vi "Setup VI for Full Monitor Res.vi"(8 "Error In":errorcluster, 11 "This VI":refnum<vi>) -> (0 "Error Out":errorcluster, 3 "VI Ref Out":refnum<vi>)   [LabVIEW 2014]
uses:
  <vilib>/Utility/miscctls.llb/LVRectTypeDef.ctl
  <vilib>/Utility/miscctls.llb/LVPointTypeDef.ctl
panel:
  out "Front Panel Window:Panel Bounds":T1
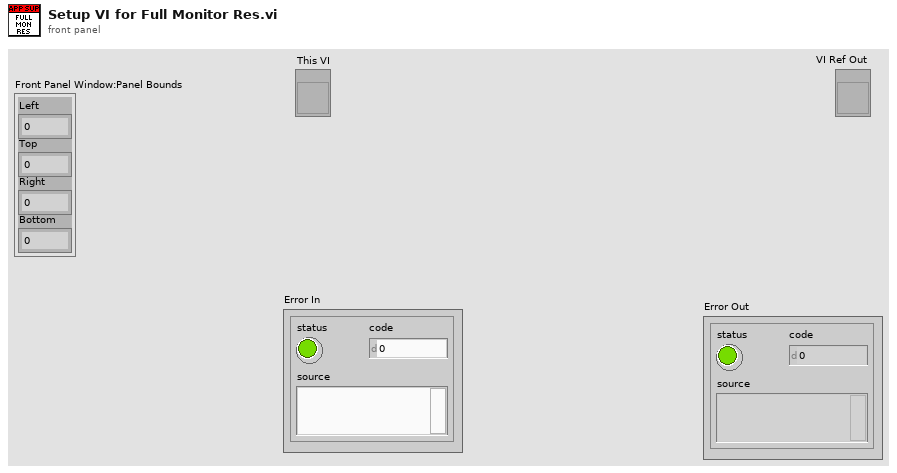
[diagram p1: front panel]
types:
  T1 = typedef "LVRectTypeDef.ctl" = cluster{"Left":i16, "Top":i16, "Right":i16, "Bottom":i16}
  T2 = typedef "LVPointTypeDef.ctl" = cluster{"Horizontal":i16, "Vertical":i16}
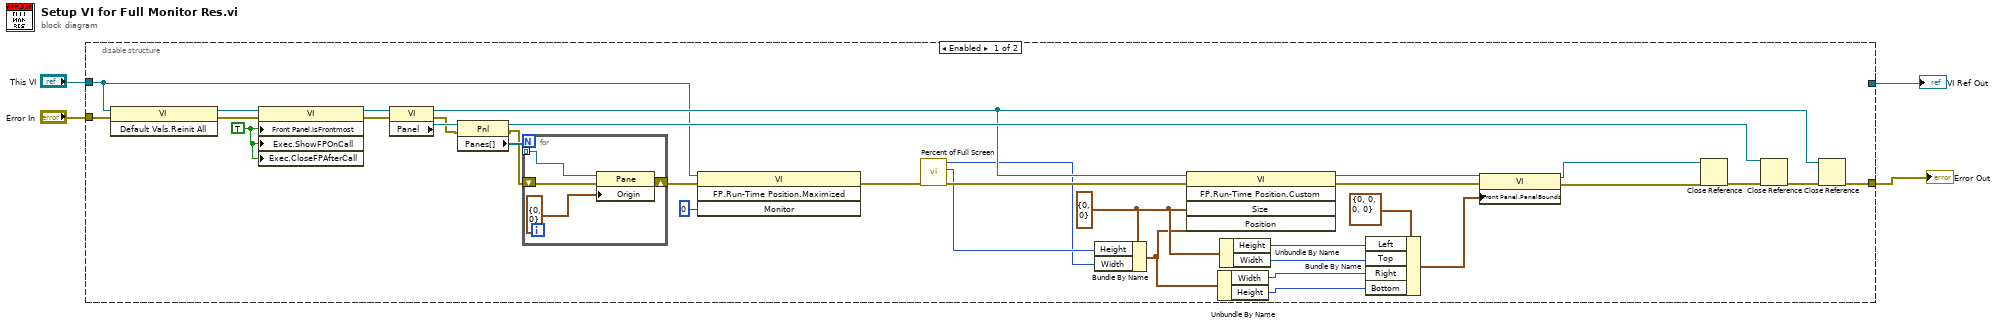
[diagram p0: block diagram]
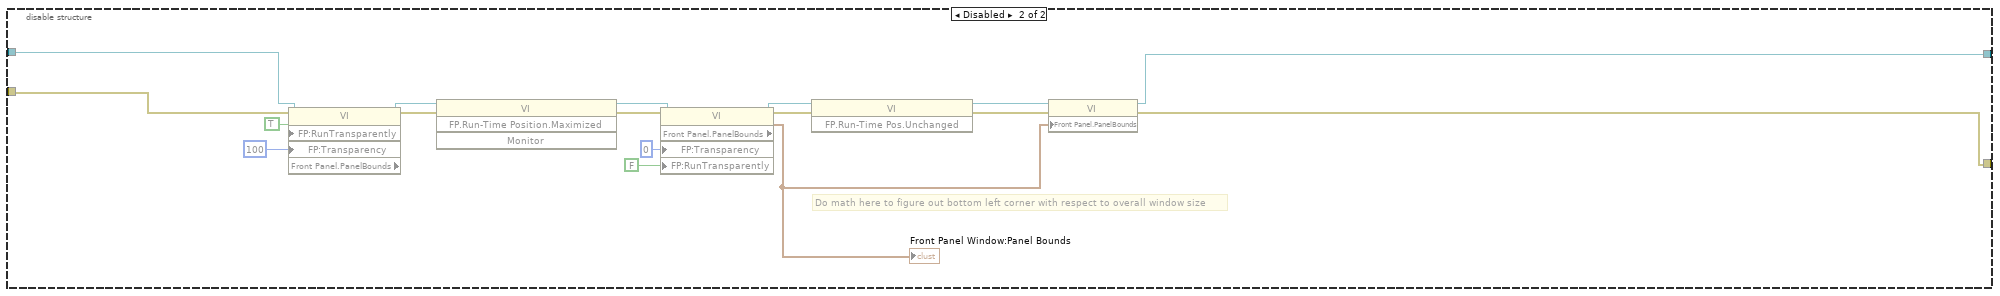
[diagram p2: hidden frame]
diagram:
  n1 = disable-structure shown="Enabled" {
    disable-tunnel: "Error In" -> [w38 w45]
    disable-tunnel: [w30 w43] -> w3
    disable-tunnel: "This VI" -> [w18 w46]
    disable-tunnel: [_ w44] -> w1
    frame Enabled {
      w24 = TRUE ("Front Panel Window:Is Frontmost")
      w11 = cluster{"Height":i16, "Width":i16} {"Height"=0, "Width"=0} ("Size")
      n2 = invoke class="VI" method="Default Vals.Reinit All"(reference=w18, error in=w38) -> (reference out=w28:refnum<vi>, error out=w25:errorcluster)  [unwired: 1 in, 1 out]
      n3 = property on="Property Node" class="VI"(reference=w28, error in=w25, "Front Panel.IsFrontmost"=w24, "Exec.ShowFPOnCall"=w24, "Exec.CloseFPAfterCall"=w24) -> (reference out=w27:refnum<vi>, error out=w26:errorcluster)
      n4 = property on="Property Node" class="VI"(reference=w27, error in=w26) -> (reference out=w29:refnum<vi>, error out=w35:errorcluster, "Panel"=w37:refnum<vi>)
      n5 = property on="Property Node" class="Pnl"(reference=w37, error in=w35) -> (reference out=w32:refnum<vi>, error out=w34:errorcluster, "Panes[]"=w36:refnum<vi>[])
      n6 = for {
        tunnel: w36 -> [w39] mode=indexing
        shift-right: [w40] -> w20
        shift-left: w34 -> [w41]
        n7 = property on="Property Node" class="Pane"(reference=w39, error in=w41, "Origin"=T2 {"Horizontal"=0, "Vertical"=0}) -> (error out=w40:errorcluster)  [unwired: 1 out]
      }
      n8 = invoke class="VI" method="FP.Run-Time Position.Maximized"(reference=w18, error in=w20, "Monitor"=i16 0) -> (error out=w17:errorcluster)  [unwired: 1 in, 3 out]
      n9 = call "Percent of Full Screen.vi"("error in (no error)"=w17) -> ("error out"=w23:errorcluster, "Bottom"=w22:i16, "Right"=w21:i16)  [unwired: 8 in]
      n10 = Bundle By Name(cluster=w11, "Height"=w22, "Width"=w21) -> (w8:cluster{"Height":i16, "Width":i16})
      n11 = invoke class="VI" method="FP.Run-Time Position.Custom"(reference=w29, error in=w23, "Size"=w11, "Position"=w8) -> (reference out=w16:refnum<vi>, error out=w15:errorcluster)  [unwired: 1 in, 3 out]
      n12 = Unbundle By Name(w8) -> ("Width"=w7:i16, "Height"=w6:i16)
      n13 = Unbundle By Name(w11) -> ("Height"=w10:i16, "Width"=w9:i16)
      n14 = Bundle By Name(cluster=T1 {"Left"=0, "Top"=0, "Right"=0, "Bottom"=0} ("Front Panel Window:Panel Bounds"), "Left"=w10, "Top"=w9, "Right"=w7, "Bottom"=w6) -> (w5:T1)
      n15 = property class="VI"(reference=w16, error in=w15, "Front Panel.PanelBounds"=w5) -> (reference out=w14:refnum<vi>, error out=w13:errorcluster)
      n16 = Close Reference(reference=w14, error in (no error)=w13) -> (error out=w33:errorcluster)
      n17 = Close Reference(reference=w32, error in (no error)=w33) -> (error out=w31:errorcluster)
      n18 = Close Reference(reference=w29, error in (no error)=w31) -> (error out=w30:errorcluster)
    }
    frame Disabled {
      # "Do math here to figure out bottom left corner with respect to overall window size"
      n19 = property class="VI" props=["FP:RunTransparently", "FP:Transparency", "Front Panel.PanelBounds"](reference=w46, error in=w45, "FP:RunTransparently"=TRUE ("Front Panel Window:Run VI Transparently"), "FP:Transparency"=u8 100 ("Front Panel Window:Transparency")) -> (reference out=w50:refnum<vi>, error out=w49:errorcluster)  [unwired: 1 out]
      n20 = invoke class="VI" method="FP.Run-Time Position.Maximized"(reference=w50, error in=w49) -> (reference out=w47:refnum<vi>, error out=w48:errorcluster)  [unwired: 2 in, 2 out]
      n21 = property class="VI"(reference=w47, error in=w48, "FP:Transparency"=u8 0 ("Front Panel Window:Transparency"), "FP:RunTransparently"=FALSE ("Front Panel Window:Run VI Transparently")) -> (reference out=w56:refnum<vi>, error out=w57:errorcluster, "Front Panel.PanelBounds"=w55:T1)
      "Front Panel Window:Panel Bounds" <- w55
      n22 = invoke class="VI" method="FP.Run-Time Pos.Unchanged"(reference=w56, error in=w57) -> (reference out=w58:refnum<vi>, error out=w59:errorcluster)  [unwired: 1 in, 1 out]
      n23 = property class="VI"(reference=w58, error in=w59, "Front Panel.PanelBounds"=w55) -> (reference out=w44:refnum<vi>, error out=w43:errorcluster)
    }
  }
  "Error Out" <- w3
  "VI Ref Out" <- w1
